vi "handle event.vi"(8 "error in":errorcluster, 10 "event":T1, 11 "module in":refnum<class "TBM module execution interface.lvclass">) -> (0 "error out":errorcluster, 3 "module out":refnum<class "TBM module execution interface.lvclass">)   [LabVIEW 2013, in "TBM module execution interface.lvclass"]
uses:
  TBM module execution interface.lvclass
  <vilib>/NI/Tag Bus/events/event.ctl
  <vilib>/NI/Tag Bus/events/data bus events.lvlib
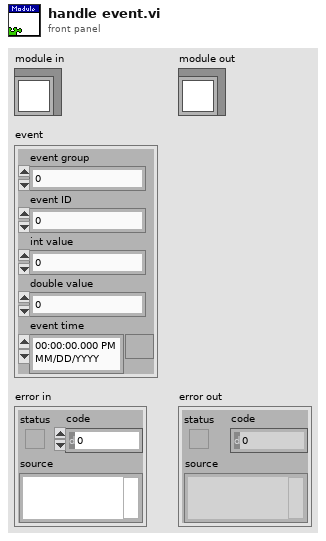
[diagram p1: front panel]
types:
  T1 = typedef "data bus events.lvlib/event.ctl" = cluster{"event group":i64, "event ID":i64, "int value":i64, "double value":dbl, "event time":timestamp}
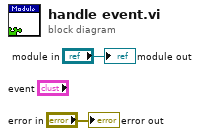
[diagram p0: block diagram]
diagram:
  "error out" <- "error in"
  "module out" <- "module in"
